vi "SavePackets.vi"(6 "DefaultFolderName(Data)":string="Data", 7 "DefaultFileExtension(FSDAT)":string="FSDAT", 11 "Packets":T1[](array[typedef]) {"MeasurementConfig"."Resolution[b]" min=4 max=16 step=1; "MeasurementConfig"."Frequency" min=1 max=10000000 step=1}) -> (0 "ErrorOut":errorcluster)   [LabVIEW 2016]
doc: "Saves packets data into a fall sensor measurement file."
uses:
  Packet.ctl
  Sample.ctl
  Reading.ctl
  MeasurementConfig.ctl
  Measurement/AccelFSRange.ctl
  Measurement/GyroFSRange.ctl
  <vilib>/addons/JSON API/JSON Object/JSON Object.lvclass
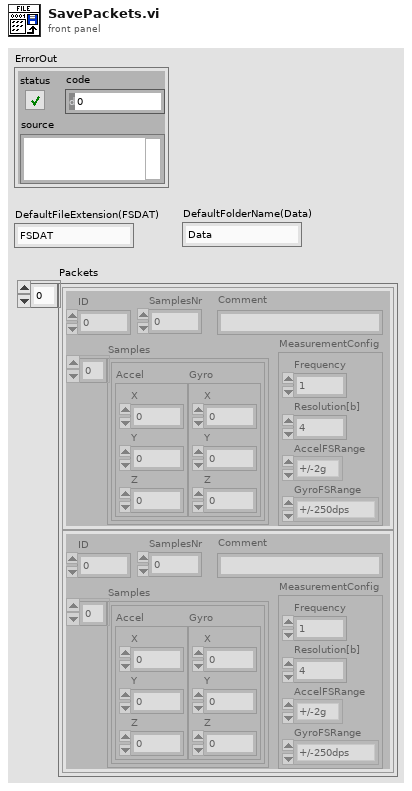
[diagram p1: front panel]
types:
  T1 = typedef "Packet.ctl" = cluster{"ID":u32, "SamplesNr":u32, "Samples":T2[], "MeasurementConfig":T4, "Comment":string}
  T2 = typedef "Sample.ctl" = cluster{"Accel":T3, "Gyro":T3}
  T3 = typedef "Reading.ctl" = cluster{"X":i16, "Y":i16, "Z":i16}
  T4 = typedef "MeasurementConfig.ctl" = cluster{"Frequency":u32, "Resolution[b]":u32, "AccelFSRange":T5, "GyroFSRange":T6}
  T5 = typedef "AccelFSRange.ctl" = enum16{"+/-2g", "+/-4g", "+/-8g", "+/-16g"}
  T6 = typedef "GyroFSRange.ctl" = enum16{"+/-250dps", "+/-500dps", "+/-1000dps", "+/-2000dps"}
  T7 = enum16{"open", "replace", "create", "open or create", "replace or create", "replace or create with confirmation"}
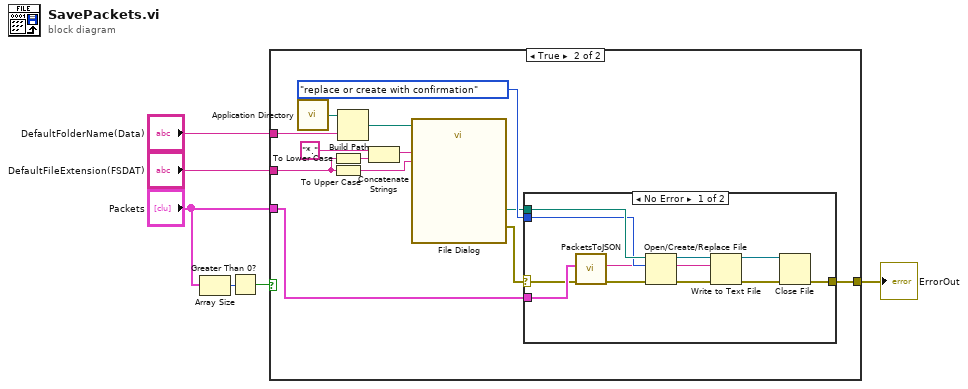
[diagram p0: block diagram]
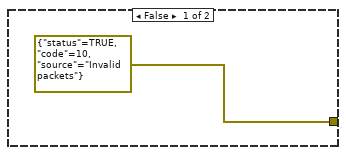
[diagram p2: hidden frame]
diagram:
  n1 = Array Size(array="Packets") -> (size(s)=w2:i32)
  n2 = Greater Than 0?(x=w2) -> (x > 0?=w1:bool)
  n3 = case shown="True" w1 {
    tunnel: "DefaultFolderName(Data)" -> [_ w19]
    tunnel: [errorcluster {"status"=TRUE, "code"=10, "source"="Invalid packets"} ("error IO") w17] -> w5
    tunnel: "DefaultFileExtension(FSDAT)" -> [_ w13]
    tunnel: "Packets" -> [_ w9]
    frame False {
    }
    frame True {
      n4 = call <vilib>:"Application Directory.vi"() -> ("Application Directory"=w20:path)
      n5 = To Lower Case(string=w13) -> (all lower case string=w15:string)
      n6 = To Upper Case(1:w13) -> (0:w16:string)
      n7 = Build Path(base path=w20, name or relative path=w19) -> (appended path=w18:path)
      n8 = Concatenate Strings("*." ("string"), w15) -> (w12:string)
      n9 = call "File Dialog"("start path"=w18, "pattern (all files)"=w12, "pattern label"=w16) -> ("selected path"=w10:path, "error out"=w8:errorcluster)  [unwired: 9 in, 2 out]
      n10 = case shown="No Error" w8 {
        selector: w8 -> [w23 w32]
        tunnel: [w31 w32] -> w17
        tunnel: T7."replace or create with confirmation" ("operation (0:open)") -> [w29 _]
        tunnel: w10 -> [w30 _]
        tunnel: w9 -> [w24 _]
        frame No Error {
          n11 = call "PacketsToJSON.vi"("ErrorIn"=w23, "Packets"=w24) -> ("ErrorOut"=w22:errorcluster, "JSONPacket"=w21:string)  [unwired: 7 in, 1 out]
          n12 = Open/Create/Replace File(file path (use dialog)=w30, error in=w22, operation (0:open)=w29) -> (refnum out=w27:refnum<file>, error out=w28:errorcluster)  [unwired: 3 in, 1 out]
          n13 = Write to Text File(file (use dialog)=w27, text=w21, error in=w28) -> (refnum out=w25:refnum<file>, error out=w26:errorcluster)  [unwired: 1 in, 1 out]
          n14 = Close File(refnum=w25, error in=w26) -> (error out=w31:errorcluster)  [unwired: 1 out]
        }
        frame Error {
        }
      }
    }
  }
  "ErrorOut" <- w5
